vi "Read Section Ref.vi"(7 "Section Name":string, 8 "error in (no error)":errorcluster, 10 "Section (Cluster)":variant, 11 "Refnum in":T1) -> (0 "error out":errorcluster, 1 "Missing key(s)":bool, 2 "Section (Cluster) out":variant, 3 "Refnum out":T1, 4 "Keys not found":string)   [LabVIEW 2024, in "Generic Config Handling.lvlib"]
doc: "This vi reads the cluster from a section in the config file. \n\nIf section name is not wired then the default is to use the name of the cluster.\n\nEach element of the cluster becomes a key, therefore it must be named, and they should be unique and not include any special characters (spaces are allowed and are replaced by_)\n\nYou cannot nest clusters and only simple datatypes are allowed. 1D and 2D arrays are allowed. They are stored as a single element with columns delimited by semicolons and rows delimited by commas. 1D arrays are stored as a single row (ie. comma delimited). \n\nEnums are stored as U32s.\n\nThe cluster wired to Section is used as the default values for the keys if they are not found. If any key is missing, missing keys is true and a list of missing keys is provided."
uses:
  Generic Config Handling.lvlib
  <vilib>/Utility/config.llb/Config Data RefNum.ctl
  <vilib>/Utility/VariantDataType/VariantType.lvlib
  <vilib>/Utility/config.llb/NI_LVConfig.lvlib
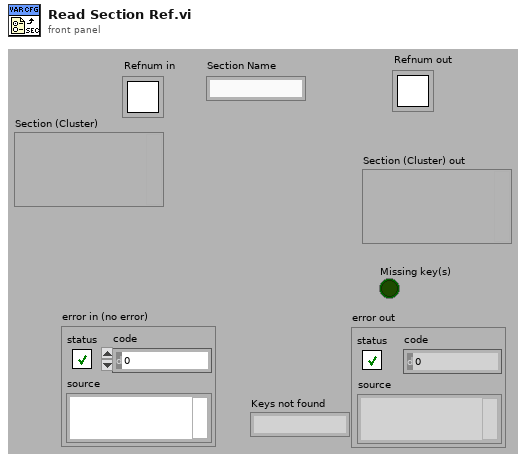
[diagram p1: front panel]
types:
  T1 = typedef "NI_LVConfig.lvlib/Config Data RefNum.ctl" = refnum<k1>
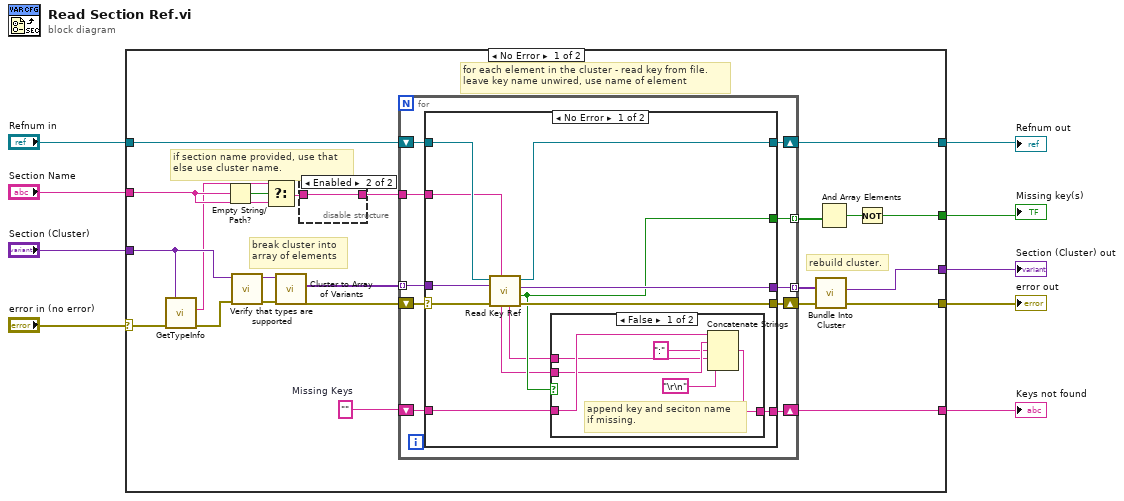
[diagram p0: block diagram]
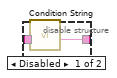
[diagram p2: hidden frame]
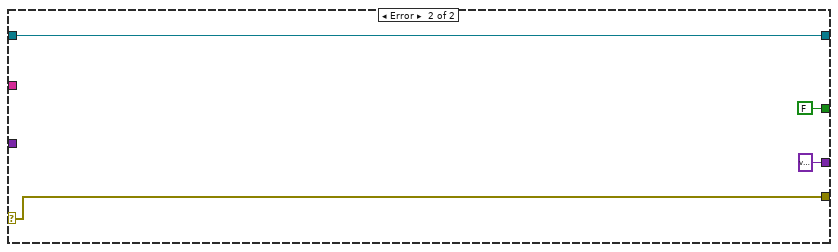
[diagram p5: hidden frame]
diagram:
  n1 = case shown="No Error" "error in (no error)" {
    selector: "error in (no error)" -> [w10 w70]
    tunnel: "Refnum in" -> [w31 w71]
    tunnel: [w30 w71] -> w8
    tunnel: "Section Name" -> [w28 _]
    tunnel: [w26 variant ("Cluster Out")] -> w6
    tunnel: [w24 w70] -> w5
    tunnel: [w20 _] -> w4
    tunnel: [w17 FALSE] -> w3
    tunnel: "Section (Cluster)" -> [w14 _]
    frame No Error {
      w21 = ""  # Missing Keys
      # "for each element in the cluster - read key from file.\nleave key name unwired, use name of element"
      # "rebuild cluster."
      # "break cluster into \narray of elements"
      # "if section name provided, use that\nelse use cluster name."
      n2 = call <vilib>:"GetTypeInfo.vi"("error in (no error)"=w10, "Variant"=w14) -> ("error out"=w13:errorcluster, "Name"=w12:string)  [unwired: 5 in, 3 out]
      n3 = Empty String/Path?(string/path=w28) -> (empty?=w29:bool)
      n4 = call "Verify that types are supported.vi"("error in"=w13, "Section (Cluster)"=w14) -> ("error out"=w15:errorcluster, "Section (Cluster)"=w16:variant)  [unwired: 8 in]
      n5 = Select(t=w12, s=w29, f=w28) -> (s? t:f=w23:string)
      n6 = call "Cluster to Array of Variants.vi"("error in (no error)"=w15, "Section (Cluster)"=w16) -> ("error out"=w11:errorcluster, "Cluster Elements"=w32:variant[])  [unwired: 7 in, 1 out]
      n7 = disable-structure shown="Enabled" {
        disable-tunnel: w23 -> [w34 w35]
        disable-tunnel: [w33 w35] -> w22
        frame Disabled {
          n8 = call "Condition String.vi"("input string"=w34) -> ("result string"=w33:string)  [unwired: 9 in, 1 out]
        }
        frame Enabled {
        }
      }
      n9 = for {
        tunnel: w22 -> [w37]
        tunnel: w32 -> [w42] mode=indexing
        shift-right: [w43] -> w25
        shift-left: w11 -> [w36]
        shift-right: [w44] -> w30
        shift-left: w31 -> [w45]
        tunnel: [w41] -> w27 mode=indexing
        tunnel: [w40] -> w19 mode=indexing
        shift-right: [w38] -> w20
        shift-left: w21 -> [w39]
        n10 = case shown="No Error" w36 {
          selector: w36 -> [w46 w67]
          tunnel: w45 -> [w56 w65]
          tunnel: [w55 w65] -> w44
          tunnel: [w54 w67] -> w43
          tunnel: w42 -> [w53 w66]
          tunnel: [w52 w66] -> w41
          tunnel: [w51 _] -> w40
          tunnel: w39 -> [w49 w64]
          tunnel: [w48 w64] -> w38
          tunnel: w37 -> [w47 _]
          frame No Error {
            n11 = call "Read Key Ref.vi"("Section"=w47, "error in (no error)"=w46, "Section Element"=w53, "Refnum in"=w56) -> ("error out"=w54:errorcluster, "found?"=w51:bool, "Variant Element Data"=w52:variant, "Refnum out"=w55:T1, "Key Name out"=w50:string)  [unwired: 3 in]
            n12 = case shown="False" w51 {
              tunnel: w50 -> [w58 _]
              tunnel: w49 -> [w62 w63]
              tunnel: [w61 w63] -> w48
              tunnel: w47 -> [w60 _]
              frame False {
                # "append key and seciton name\nif missing."
                n13 = Concatenate Strings(w62, w60, ":" ("string"), w58, "\r\n") -> (w61:string)
              }
              frame True {
              }
            }
          }
          frame Error {
          }
        }
      }
      n14 = call "Bundle Into Cluster.vi"("error in"=w25, "Cluster Elements in"=w27) -> ("error out"=w24:errorcluster, "Cluster Out"=w26:variant)  [unwired: 8 in]
      n15 = And Array Elements(Boolean array=w19) -> (logical AND=w18:bool)
      n16 = Not(x=w18) -> (.not. x?=w17:bool)
    }
    frame Error {
    }
  }
  "Refnum out" <- w8
  "error out" <- w5
  "Section (Cluster) out" <- w6
  "Keys not found" <- w4
  "Missing key(s)" <- w3
